vi "Get SMO Name.vi"(8 "error in (no error)":errorcluster, 11 "instrument.PPMS3 in":refnum<class "instrument.OptiCool.lvclass">) -> (0 "error out":errorcluster, 2 "SMO Name":string, 3 "instrument.PPMS3 out":refnum<class "instrument.OptiCool.lvclass">)   [LabVIEW 2019, in "instrument.OptiCool.lvclass"]
uses:
  instrument.OptiCool.lvclass
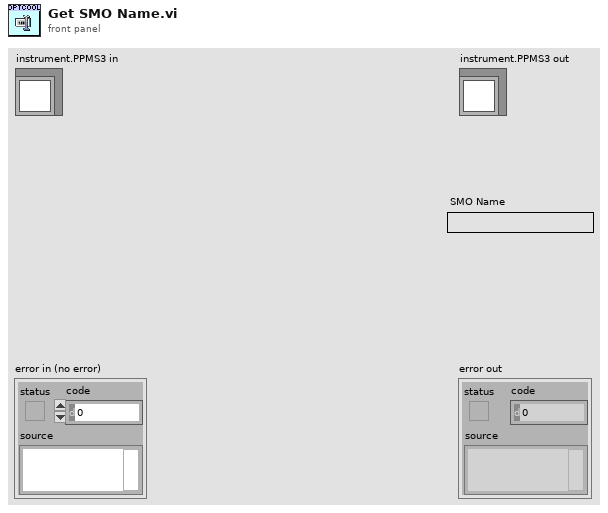
[diagram p1: front panel]
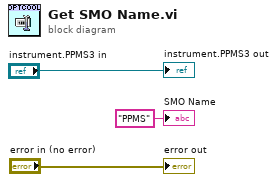
[diagram p0: block diagram]
diagram:
  "error out" <- "error in (no error)"
  "instrument.PPMS3 out" <- "instrument.PPMS3 in"
  "SMO Name" <- "PPMS" ("SMO Name")
